vi "RefnumToLableValue.vi"(1 "Ctl Refnum":refnum<vi>) -> (0 "Control Lable Value String":string)   [LabVIEW 2020]
doc: "It will convert Numeric, Boolean, String controls to a fixed length text row by getting the control's refnum as input. The text row included the label of the control and its value. It is used to used the used control values as a reference to future or futher used and anlysis."
uses:
  <vilib>/Utility/Data Type/NI_Data Type.lvlib
panel:
  # "This VI Will not work for Boolean with the latch mechanics"
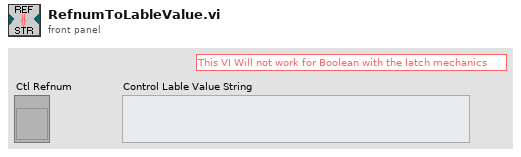
[diagram p1: front panel]
types:
  T1 = typedef "NI_Data Type.lvlib/Data Type.ctl" = enum8{"Invalid Type", "Void", "I8", "I16", "I32", "I64", "U8", "U16", "U32", "U64", "Single Float", "Double Float", "Extended Float", "Single Complex", "Double Complex", "Extended Complex", "Enum U8", "Enum U16", "Enum U32", "Enum U64", "Single Float With Unit", "Double Float With Unit", "Extended Float With Unit", "Single Complex with Unit", "Double Complex with Unit", "Extended Complex with Unit", "Boolean", "String", "Path", "Picture", "Tag", "Array", "Cluster", "Variant", "LV Variant", "Waveform", "Timestamp", "Digital Waveform", "Digital Data", "ExpressData", "Refnum", "External Data", "VI", "Poly VI", "LabVIEW Class Instance", "Fixed Point", "Set Collection", "Map Collection"}
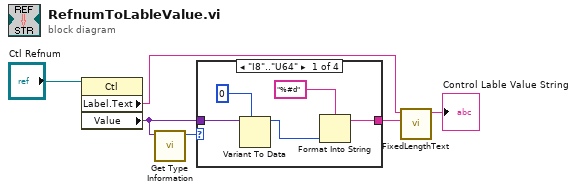
[diagram p0: block diagram]
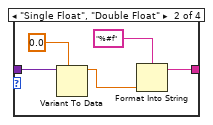
[diagram p2: hidden frame]
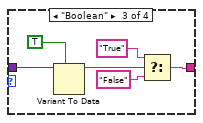
[diagram p3: hidden frame]
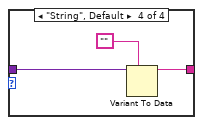
[diagram p4: hidden frame]
diagram:
  n1 = property class="Ctl"(reference="Ctl Refnum") -> ("Label.Text"=w5:string, "Value"=w2:variant)  [unwired: 1 in, 2 out]
  n2 = call <vilib>:"Get Type Information.vi"("variant"=w2) -> ("type"=w3:T1)  [unwired: 6 in, 4 out]
  n3 = case shown="\"I8\"..\"U64\"" w3 {
    tunnel: w2 -> [w11 w16 w22 w25]
    tunnel: [w8 w12 w17 w23] -> w1
    frame "I8".."U64" {
      n4 = Variant To Data(type=0, Variant=w11) -> (data=w7:i32)  [unwired: 1 in, 1 out]
      n5 = Format Into String(format string="%#d", w7) -> (resulting string=w8:string)  [unwired: 2 in, 1 out]
    }
    frame "Single Float", "Double Float" {
      n6 = Variant To Data(type=0.0, Variant=w16) -> (data=w13:dbl)  [unwired: 1 in, 1 out]
      n7 = Format Into String(format string="%#f", w13) -> (resulting string=w12:string)  [unwired: 2 in, 1 out]
    }
    frame "Boolean" {
      n8 = Variant To Data(type=TRUE, Variant=w22) -> (data=w20:bool)  [unwired: 1 in, 1 out]
      n9 = Select(t="True", s=w20, f="False") -> (s? t:f=w17:string)
    }
    frame "String", Default {
      n10 = Variant To Data(type="", Variant=w25) -> (data=w23:string)  [unwired: 1 in, 1 out]
    }
  }
  n11 = call "FixedLengthText.vi"("Value"=w1, "Label"=w5) -> ("Lable Value String"=→"Control Lable Value String":string)  [unwired: 9 in]
